vi "thorlabs_handle_error.vi"(8 "error in (no error)":errorcluster, 11 "thorlabs_panel in":refnum<class "thorlabs_panel.lvclass">) -> (0 "error out":errorcluster, 3 "thorlabs_panel out":refnum<class "thorlabs_panel.lvclass">)   [LabVIEW 2015, in "thorlabs_panel.lvclass"]
uses:
  thorlabs_panel.lvclass
  thorlabs_panel.lvclass/thorlabs_panel.ctl
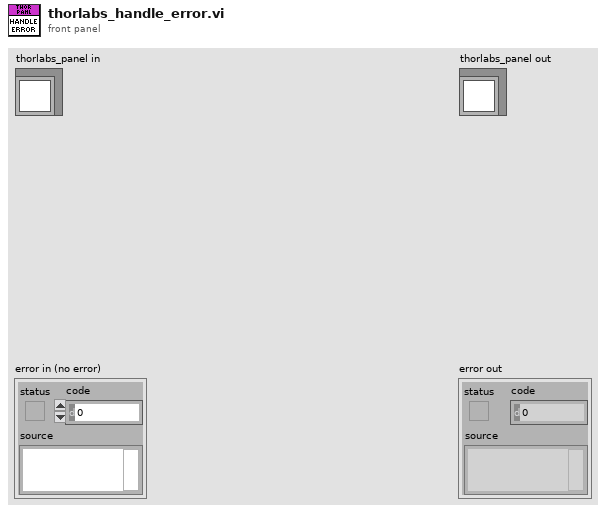
[diagram p1: front panel]
types:
  T1 = typedef "thorlabs_events.ctl" = cluster{"mcl_status":refnum<user-event>, "piezo_positions":refnum<user-event>}
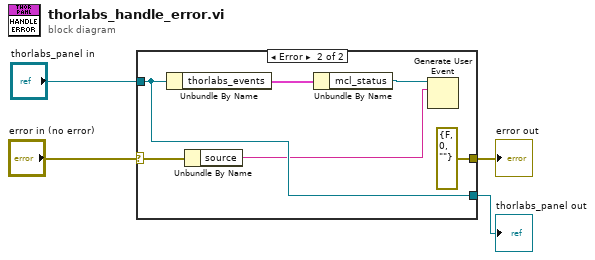
[diagram p0: block diagram]
diagram:
  n1 = case shown="Error" "error in (no error)" {
    selector: "error in (no error)" -> [w5 w12]
    tunnel: [w5 errorcluster {"status"=FALSE, "code"=0, "source"=""} ("error IO")] -> w3
    tunnel: [w6 w11] -> w1
    tunnel: "thorlabs_panel in" -> [w6 w11]
    frame No Error {
    }
    frame Error {
      n2 = Unbundle By Name(w11) -> ("thorlabs_events"=w10:T1)
      n3 = Unbundle By Name(w12) -> ("source"=w8:string)
      n4 = Unbundle By Name(w10) -> ("mcl_status"=w9:refnum<user-event>)
      n5 = Generate User Event(user event=w9, event data cluster=w8) -> ()  [unwired: 2 in, 2 out]
    }
  }
  "error out" <- w3
  "thorlabs_panel out" <- w1
